vi "simx Auxiliary Console Open.vi"(0 "clientID":i32, 1 "title":string, 2 "maxLines":i32, 3 "mode":i32, 4 "position":i32, 5 "size":i32, 6 "textColor":sgl, 7 "error in (no error)":errorcluster, 8 "backgroundColor":sgl, 9 "consoleHandle":i32, 10 "operationMode":i32) -> (18 "backgroundColor out":sgl, 19 "consoleHandle out":i32, 20 "function return":i32, 24 "position out":i32, 25 "size out":i32, 26 "textColor out":sgl, 27 "error out":errorcluster)   [LabVIEW 2019, in "PXL_V-REP.lvlib"]
doc: "EXTAPI_DLLEXPORT simxInt simxAuxiliaryConsoleOpen(simxInt clientID,const simxChar* title,simxInt maxLines,simxInt mode,simxInt* position,simxInt* size,simxFloat* textColor,simxFloat* backgroundColor,simxInt* consoleHandle,simxInt operationMode);"
uses:
  PXL_V-REP.lvlib
  <userlib>/V-REP/remoteApi.dll
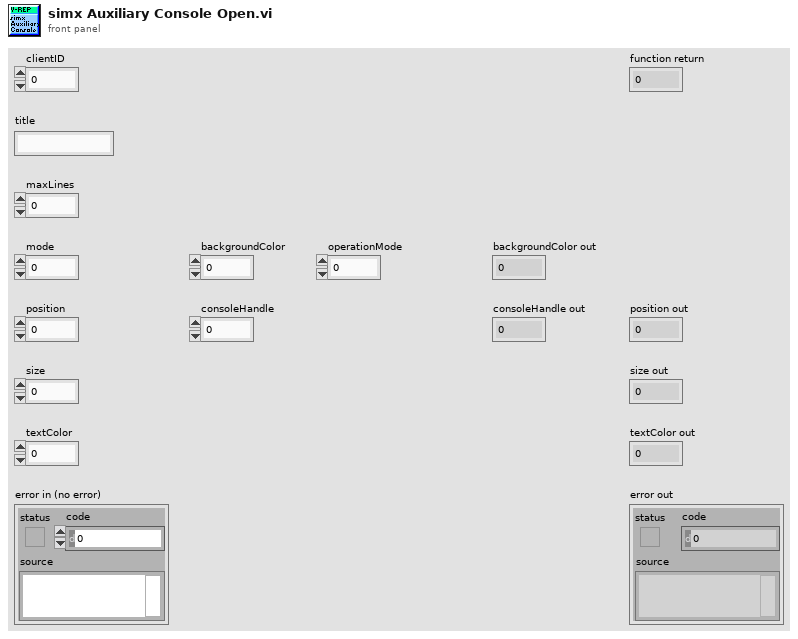
[diagram p1: front panel]
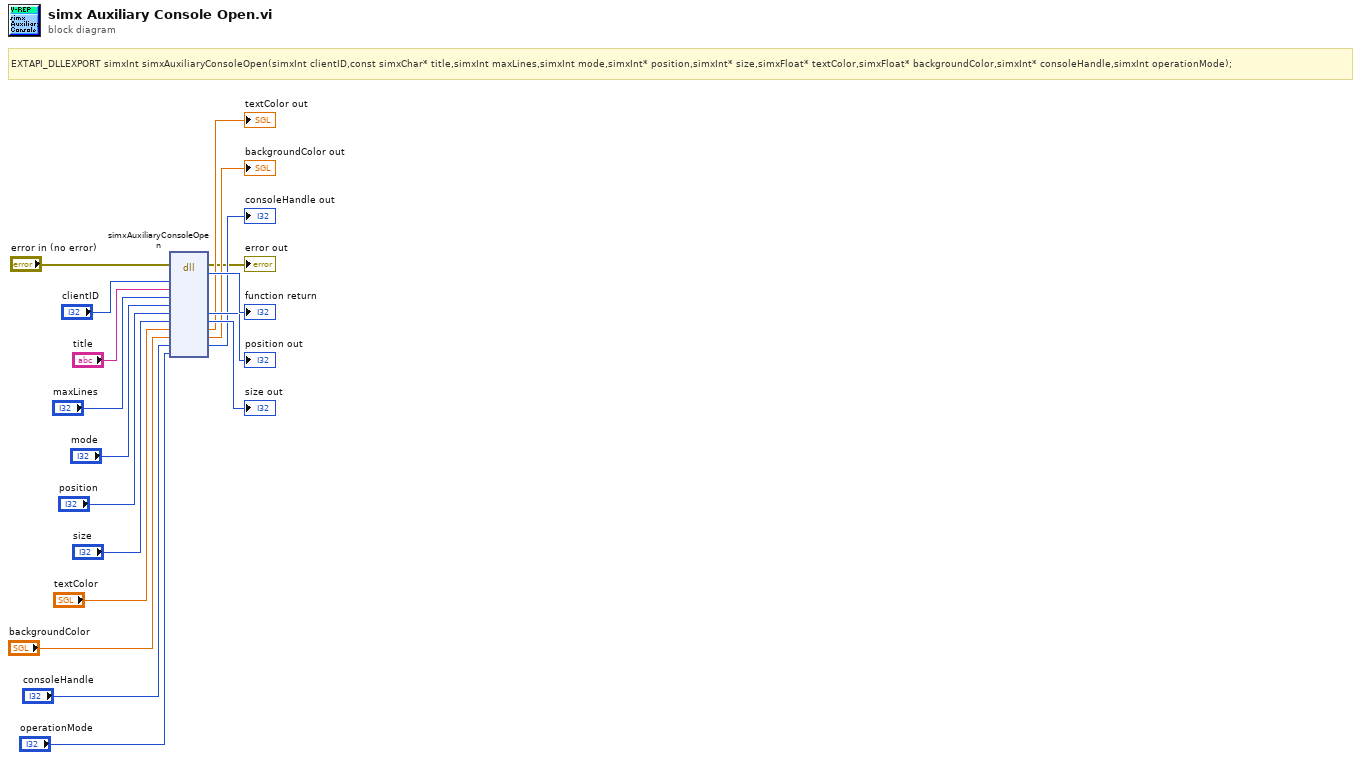
[diagram p0: block diagram]
diagram:
  # "EXTAPI_DLLEXPORT simxInt simxAuxiliaryConsoleOpen(simxInt clientID,const simxChar* title,simxInt maxLines,simxInt mode,simxInt* position,simxInt* size,simxFloat* textColor,simxFloat* backgroundColor,simxInt* consoleHandle,simxInt operationMode);"
  n1 = dll-call lib="C:/Program Files (x86)/National Instruments/LabVIEW 2019/user.lib/V-REP/remoteApi.*" fn="simxAuxiliaryConsoleOpen"(error in="error in (no error)", "clientID"="clientID", "title"="title", "maxLines"="maxLines", "mode"="mode", "position"="position", "size"="size", "textColor"="textColor", "backgroundColor"="backgroundColor", "consoleHandle"="consoleHandle", "operationMode"="operationMode") -> (error out=→"error out":errorcluster, →"function return":i32, "position"=→"position out":i32, "size"=→"size out":i32, "textColor"=→"textColor out":sgl, "backgroundColor"=→"backgroundColor out":sgl, "consoleHandle"=→"consoleHandle out":i32)  [unwired: 7 in, 1 out]
